vi "rotate polygon.vi"(7 "Anticlockwise rotations [0-3] (0)":i32, 10 "Polygon Corners in":cluster{"x":dbl, "y":dbl}[](array[cluster])=[{"x"=9.857142857142858, "y"=0.0}, {"x"=23.0, "y"=0.0}, {"x"=23.0, "y"=150.0}, {"x"=0.0, "y"=150.0}, {"x"=0.0, "y"=100.0}, {"x"=9.857142857142858, "y"=100.0}, {"x"=9.857142857142858, "y"=0.0}]) -> (2 "Rotated Polygone Corners out":cluster{"x":dbl, "y":dbl}[](array[cluster])=[{"x"=9.857142857142858, "y"=0.0}, {"x"=23.0, "y"=0.0}, {"x"=23.0, "y"=150.0}, {"x"=0.0, "y"=150.0}, {"x"=0.0, "y"=100.0}, {"x"=9.857142857142858, "y"=100.0}, {"x"=9.857142857142858, "y"=0.0}])   [LabVIEW 2020, in "midi-ui.lvclass"]
uses:
  midi-ui.lvclass
  midi-ui.lvclass/midi-ui.ctl
  <vilib>/ptbypt/NI_PtbyPt.lvlib
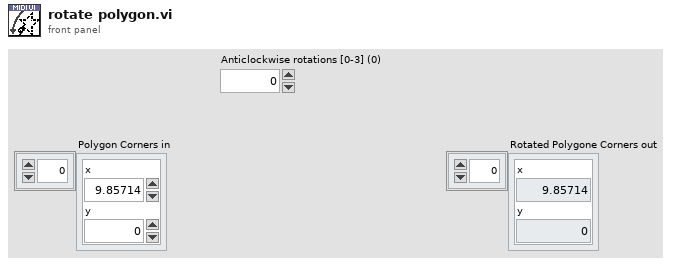
[diagram p1: front panel]
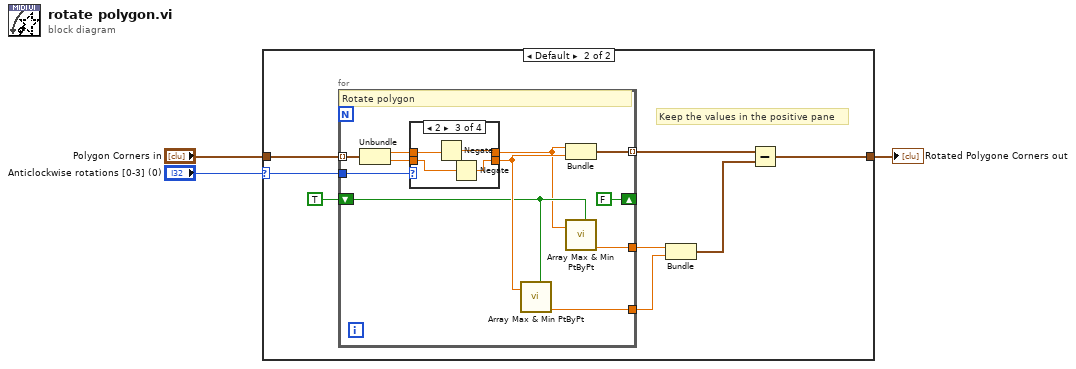
[diagram p0: block diagram]
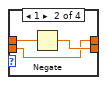
[diagram p4: hidden frame]
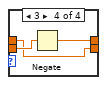
[diagram p5: hidden frame]
diagram:
  n1 = case shown="Default" "Anticlockwise rotations [0-3] (0)" {
    selector: "Anticlockwise rotations [0-3] (0)" -> [_ w5]
    tunnel: "Polygon Corners in" -> [w4 w12]
    tunnel: [w4 w11] -> w2
    frame 0 {
    }
    frame Default {
      # "Keep the values in the positive pane"
      n2 = for {
        tunnel: w12 -> [w23] mode=indexing
        tunnel: [w22] -> w10 mode=indexing
        tunnel: [w19] -> w8
        tunnel: [w18] -> w7
        shift-right: [FALSE] -> _
        shift-left: TRUE -> [w17]
        tunnel: w5 -> [w15]
        # "Rotate polygon"
        n3 = Unbundle(w23) -> ("x"=w21:dbl, "y"=w13:dbl)
        n4 = case shown="2" w15 {
          tunnel: w21 -> [w25 w28 w32 w33]
          tunnel: [w24 w27 w29 w33] -> w20
          tunnel: [w25 w26 w31 w34] -> w14
          tunnel: w13 -> [w24 w26 w30 w35]
          frame Default {
          }
          frame 1 {
            n5 = Negate(x=w28) -> (-x=w27:dbl)
          }
          frame 2 {
            n6 = Negate(x=w32) -> (-x=w31:dbl)
            n7 = Negate(x=w30) -> (-x=w29:dbl)
          }
          frame 3 {
            n8 = Negate(x=w35) -> (-x=w34:dbl)
          }
        }
        n9 = call <vilib>:"Array Max & Min PtByPt.vi"("input data point"=w20, "initialize"=w17) -> ("min value"=w18:dbl)  [unwired: 1 in, 4 out]
        n10 = Bundle("y"=w14, "x"=w20) -> (w22:cluster{"y":dbl, "x":dbl})  [unwired: 1 in]
        n11 = call <vilib>:"Array Max & Min PtByPt.vi"("input data point"=w14, "initialize"=w17) -> ("min value"=w19:dbl)  [unwired: 1 in, 4 out]
      }
      n12 = Bundle("min value"=w8, "min value"=w7) -> (w6:cluster{"min value":dbl, "min value":dbl})  [unwired: 1 in]
      n13 = Subtract(x=w10, y=w6) -> (x-y=w11:cluster{dbl, dbl}[])
    }
  }
  "Rotated Polygone Corners out" <- w2
